vi "ALTS-2015 Check Error when Reading Test Results from DB.vi"(8 "error in":errorcluster, 11 "Station Enum":T1) -> (0 "error out":errorcluster)   [LabVIEW 2013]
doc: "Copyright © 2005, Soliton Technologies.\nAll rights reserved."
uses:
  Controls/ALTS-2015 Station Cluster.ctl
  Controls/ALTS-2015 LV2GBL Options.ctl
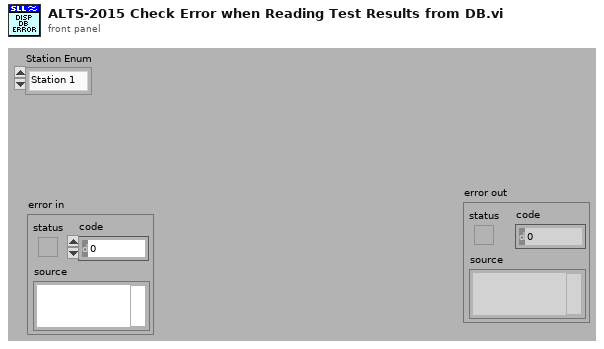
[diagram p1: front panel]
types:
  T1 = typedef "ALTS-2015 Station Cluster.ctl" = enum16{"Station 1", "Station 2", "Station 3", "Station 4"}
  T2 = typedef "ALTS-2015 LV2GBL Options.ctl" = enum16{"Read all", "Write all"}
  T3 = typedef "ALTS-2015 INI Configuration Cluster.ctl" = cluster{"Application":cluster{"Rerun Count":i32, "Workorder No":string, "PLC Scanner":bool, "Time Delay to Restart(mins)":dbl}, "Station Details":cluster{"Sensor Name 1":string, "Sensor Name 2":string, "Sensor Name 3":string, "Sensor Name 4":string, "Station1 Enable":bool, "Station2 Enable":bool, "Station3 Enable":bool, "Station4 Enable":bool}, "Database":cluster{"Database Connection Link":path, "Result Procedure":string, "User":string, "Password":string, "Prompt":bool, "Station 1 LT Result DB DSN Path":path, "Station 2 LT Result DB DSN Path":path, "Station 3 LT Result DB DSN Path":path, "Station 4 LT Result DB DSN Path":path, "AirLeakTestResult Procedure":string, "Serial Details Procedure":string}, "Simulation":cluster{"Simulate DAQ Hardware":bool, "Simulate Result DB Write":bool, "Simulate Scanner":bool, "Simulate OPC":bool, "Simulate Serial Details DB":bool, "Simulate Result DB":bool, "Simulate Scanner DB Path":path, "Simulate Serial Details DB Path":path, "Simulate Result DB Path":path}, "Barcode Scanner1":cluster{"Scanner IP":string, "Scanner Port":u16, "#Bytes to Read":i32, "Timeout_ms":i32}, "Barcode Scanner2":cluster{"Enabled?":bool, "Scanner IP":string, "Scanner Port":u16, "#Bytes to Read":i32}}
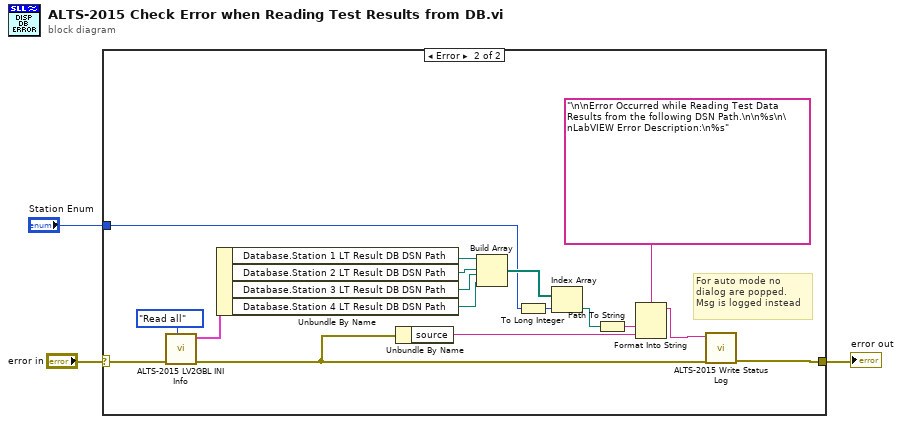
[diagram p0: block diagram]
diagram:
  n1 = case shown="Error" "error in" {
    selector: "error in" -> [w4 w18]
    tunnel: [w4 w21] -> w2
    tunnel: "Station Enum" -> [_ w8]
    frame No Error {
      # "Point Comment"
      # "Important point"
      # "Description"
    }
    frame Error {
      # "For auto mode no\ndialog are popped.\nMsg is logged instead"
      n2 = call "ALTS-2015 LV2GBL INI Info.vi"("Options"=ALTS-2015_LV2GBL_Options."Read all", "error in"=w18) -> ("error out"=w17:errorcluster, "Configuration Cluster Out"=w19:T3)  [unwired: 8 in]
      n3 = Unbundle By Name(w19) -> ("Database.Station 1 LT Result DB DSN Path"=w13:path, "Database.Station 2 LT Result DB DSN Path"=w12:path, "Database.Station 3 LT Result DB DSN Path"=w11:path, "Database.Station 4 LT Result DB DSN Path"=w10:path)
      n4 = Unbundle By Name(w17) -> ("source"=w20:string)
      n5 = Build Array(w13, w12, w11, w10) -> (w9:path[])
      n6 = To Long Integer(number=w8) -> (32bit integer=w6:i32)
      n7 = Index Array(array=w9, index=w6) -> (element=w7:path)
      n8 = Path To String(path=w7) -> (string=w16:string)
      n9 = Format Into String(format string="\n\nError Occurred while Reading Test Data Results from the following DSN Path.\n\n%s\n\nLabVIEW Error Description:\n%s", w16, w20) -> (resulting string=w14:string)  [unwired: 2 in, 1 out]
      n10 = call "ALTS-2015 Write Status Log.vi"("error in (no error)"=w17, "Status Input"=w14) -> ("error out"=w21:errorcluster)  [unwired: 9 in]
    }
  }
  "error out" <- w2
